vi "Update Cart Status.vi"(7 "Selection":T2, 8 "error in (no error)":errorcluster, 9 "String":string, 10 "Array":bool[](array[boolean]), 11 "FP":T1) -> (0 "error out":errorcluster)   [LabVIEW 2018]
uses:
  status update.ctl
  Main Refs.ctl
  Hardware/Tecan/Pump Config.ctl
  Vacuum Specs.ctl
  Timing Specs.ctl
  Cartridges.ctl
  Cartridge Status.ctl
  Commands.ctl
  Lib/Time/Wells.ctl
  Lib/Time/Bottles.ctl
  Process State.ctl
  Vacuum Test.ctl
panel:
  # "Tecan Pump"
  # "Vacuum"
  # "General"
  # "Timing"
  # "Protocol"
  # "Zaber"
  # "NFC Reader 1"
  # "NFC  Reader 2"
  # "NFC Reader 3"
  # "NFC Reader 4"
  # "System"
  # "Cartridge Utitlies"
  # "Wells"
  # "times"
  # "from"
  # "State Machine"
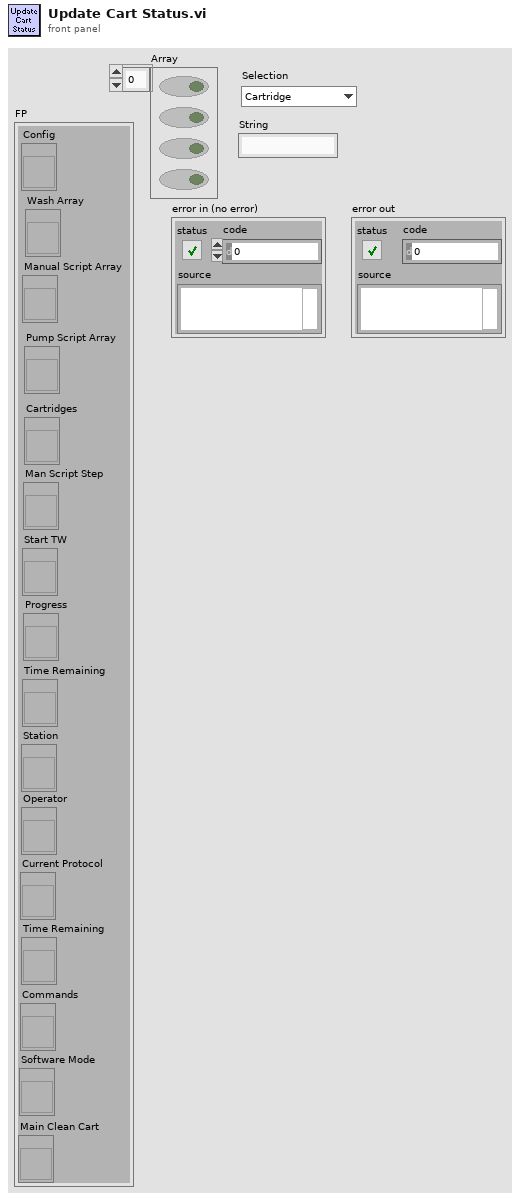
[diagram p1: front panel]
types:
  T1 = typedef "Main Refs.ctl" = cluster{"Config":refnum<vi>, "Wash Array":refnum<vi>, "Manual Script Array":refnum<vi>, "Pump Script Array":refnum<vi>, "Cartridges":refnum<vi>, "Man Script Step":refnum<vi>, "Start TW":refnum<vi>, "Progress":refnum<vi>, "Time Remaining":refnum<vi>, "Station":refnum<vi>, "Operator":refnum<vi>, "Current Protocol":refnum<vi>, "Time Remaining":refnum<vi>, "Commands":refnum<vi>, "Software Mode":refnum<vi>, "Main Clean Cart":refnum<vi>}
  T2 = typedef "status update.ctl" = enum16{"Cartridge", "Main Status", "Reagent"}
  T3 = typedef "Cartridges.ctl" = cluster{"Cartridge 1":T4, "Cartridge 2":T4, "Cartridge 3":T4, "Cartridge 4":T4, "Current Status":string}
  T4 = typedef "Cartridge Status.ctl" = cluster{"Serial Number":string, "Reagent":string, "Cart Status":string, "Inserted":bool, "Eject":bool}
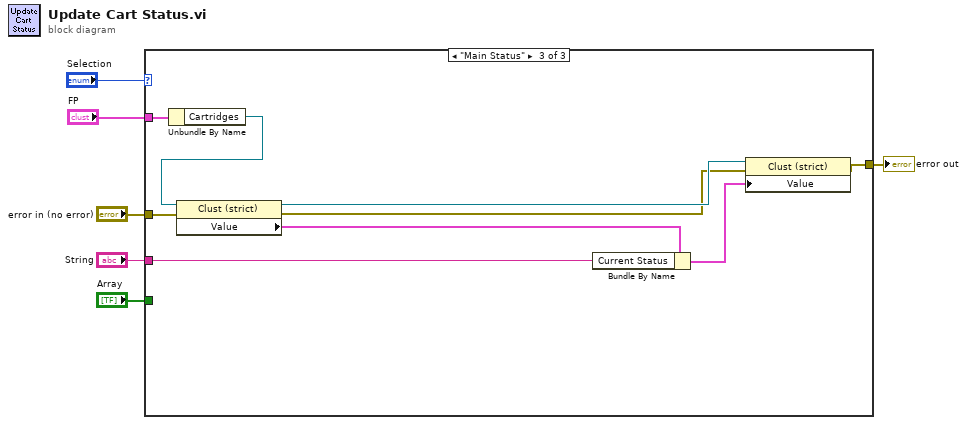
[diagram p0: block diagram]
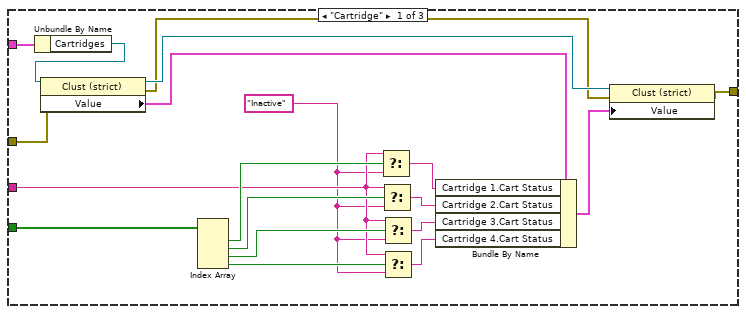
[diagram p2: hidden frame]
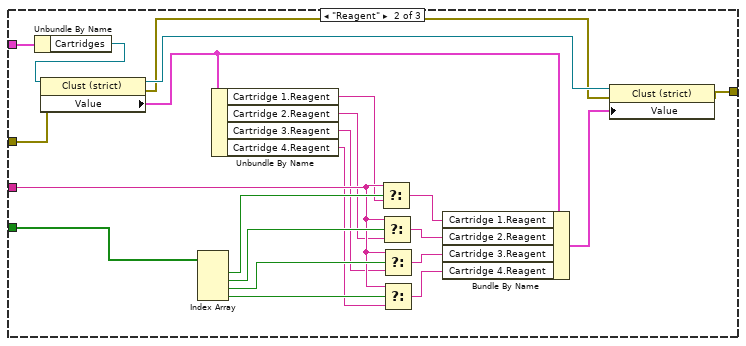
[diagram p3: hidden frame]
diagram:
  n1 = case shown="\"Main Status\"" "Selection" {
    tunnel: "Array" -> [w25 w47 _]
    tunnel: "String" -> [w20 w42 w50]
    tunnel: "error in (no error)" -> [w12 w35 w53]
    tunnel: [w10 w33 w51] -> w3
    tunnel: "FP" -> [w8 w32 w49]
    frame "Cartridge" {
      w9 = "Inactive" ("f")
      n2 = Unbundle By Name(w8) -> ("Cartridges"=w7:refnum<vi>)
      n3 = property class="Clust (strict)"(reference=w7, error in=w12) -> (reference out=w14:refnum<vi>, error out=w11:errorcluster, "Value"=w19:T3)
      n4 = Index Array(array=w25) -> (element #1=w24:bool, element #2=w23:bool, element #3=w22:bool, element #4=w21:bool)  [unwired: 4 in]
      n5 = Select(t=w20, s=w24, f=w9) -> (s? t:f=w18:string)
      n6 = Select(t=w20, s=w23, f=w9) -> (s? t:f=w17:string)
      n7 = Select(t=w20, s=w22, f=w9) -> (s? t:f=w16:string)
      n8 = Select(t=w20, s=w21, f=w9) -> (s? t:f=w15:string)
      n9 = Bundle By Name(cluster=w19, "Cartridge 1.Cart Status"=w18, "Cartridge 2.Cart Status"=w17, "Cartridge 3.Cart Status"=w16, "Cartridge 4.Cart Status"=w15) -> (w13:T3)
      n10 = property class="Clust (strict)"(reference=w14, error in=w11, "Value"=w13) -> (error out=w10:errorcluster)  [unwired: 1 out]
    }
    frame "Reagent" {
      n11 = Unbundle By Name(w32) -> ("Cartridges"=w31:refnum<vi>)
      n12 = property class="Clust (strict)"(reference=w31, error in=w35) -> (reference out=w37:refnum<vi>, error out=w34:errorcluster, "Value"=w30:T3)
      n13 = Index Array(array=w47) -> (element #1=w46:bool, element #2=w45:bool, element #3=w44:bool, element #4=w43:bool)  [unwired: 4 in]
      n14 = Unbundle By Name(w30) -> ("Cartridge 1.Reagent"=w29:string, "Cartridge 2.Reagent"=w28:string, "Cartridge 3.Reagent"=w27:string, "Cartridge 4.Reagent"=w26:string)
      n15 = Select(t=w42, s=w46, f=w29) -> (s? t:f=w41:string)
      n16 = Select(t=w42, s=w45, f=w28) -> (s? t:f=w40:string)
      n17 = Select(t=w42, s=w44, f=w27) -> (s? t:f=w39:string)
      n18 = Select(t=w42, s=w43, f=w26) -> (s? t:f=w38:string)
      n19 = Bundle By Name(cluster=w30, "Cartridge 1.Reagent"=w41, "Cartridge 2.Reagent"=w40, "Cartridge 3.Reagent"=w39, "Cartridge 4.Reagent"=w38) -> (w36:T3)
      n20 = property class="Clust (strict)"(reference=w37, error in=w34, "Value"=w36) -> (error out=w33:errorcluster)  [unwired: 1 out]
    }
    frame "Main Status" {
      n21 = Unbundle By Name(w49) -> ("Cartridges"=w48:refnum<vi>)
      n22 = property class="Clust (strict)"(reference=w48, error in=w53) -> (reference out=w55:refnum<vi>, error out=w52:errorcluster, "Value"=w56:T3)
      n23 = Bundle By Name(cluster=w56, "Current Status"=w50) -> (w54:T3)
      n24 = property class="Clust (strict)"(reference=w55, error in=w52, "Value"=w54) -> (error out=w51:errorcluster)  [unwired: 1 out]
    }
  }
  "error out" <- w3
